vi "change_color_palette_hot_cold_pixels.vi"(8 "error in (no error)":errorcluster, 10 "raw channel index":i32, 11 "DisplayDL090216 in":refnum<class "DisplayDL090216.lvclass">) -> (0 "error out":errorcluster, 3 "DisplayDL090216 out":refnum<class "DisplayDL090216.lvclass">)   [LabVIEW 2010, in "DisplayDL090216.lvclass"]
uses:
  DisplayDL090216.lvclass
  DisplayDL090216.lvclass/DisplayDL090216.ctl
  common/classes/ColorOverlay/ColorOverlay/ColorOverlay.lvclass
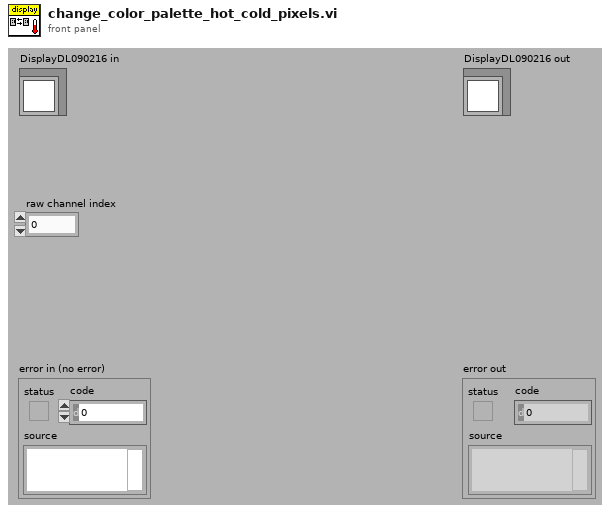
[diagram p1: front panel]
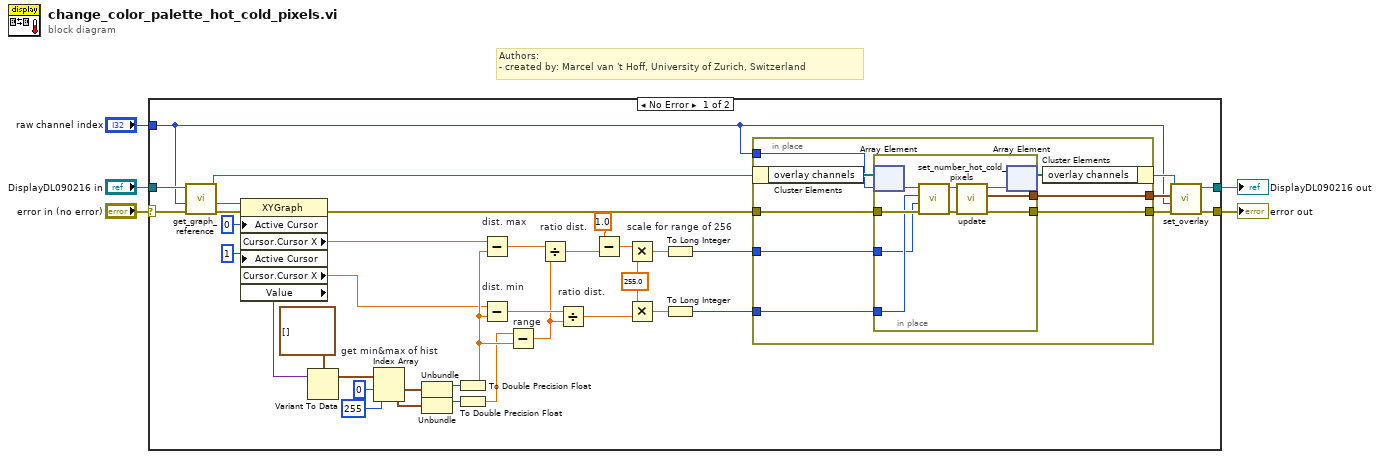
[diagram p0: block diagram]
diagram:
  # "Authors: \n- created by: Marcel van 't Hoff, University of Zurich, Switzerland"
  n1 = case shown="No Error" "error in (no error)" {
    selector: "error in (no error)" -> [w16 w63]
    tunnel: [w6 w63] -> w1
    tunnel: [w7 w62] -> w2
    tunnel: "DisplayDL090216 in" -> [w21 w62]
    tunnel: "raw channel index" -> [w8 _]
    frame No Error {
      w40 = 255.0
      n2 = call-dynamic "get_graph_reference.vi"("error in (no error)"=w16, "raw channel index"=w8, "DisplayDL090216 in"=w21) -> ("error out"=w20:errorcluster, "histogram reference out"=w19:refnum<vi>, "DisplayDL090216 out"=w10:refnum<class "DisplayDL090216.lvclass">)  [unwired: 6 in]
      n3 = property class="XYGraph"(reference=w19, error in=w20, "Active Cursor"=u32 0, "Active Cursor"=u32 1) -> (error out=w15:errorcluster, "Cursor.Cursor X"=w13:dbl, "Cursor.Cursor X"=w14:dbl, "Value"=w35:variant)  [unwired: 1 out]
      n4 = Variant To Data(Variant=w35, type=cluster{i32, u32}[] [] ("histogram out")) -> (data=w34:cluster{i32, u32}[])  [unwired: 1 in, 1 out]
      n5 = Index Array "get min&max of hist"(array=w34, index #1=0 ("index"), index #2=255 ("index")) -> (element #1=w33:cluster{i32, u32}, element #2=w32:cluster{i32, u32})
      n6 = Unbundle(w33) -> (w29:i32)  [unwired: 1 out]
      n7 = Unbundle(w32) -> (w28:i32)  [unwired: 1 out]
      n8 = To Double Precision Float(number=w29) -> (double precision float=w27:dbl)
      n9 = To Double Precision Float(number=w28) -> (double precision float=w26:dbl)
      n10 = Subtract "dist. max"(x=w13, y=w27) -> (x-y=w43:dbl)
      n11 = Subtract "dist. min"(x=w14, y=w27) -> (x-y=w44:dbl)
      n12 = Subtract "range"(x=w26, y=w27) -> (x-y=w42:dbl)
      n13 = Divide "ratio dist."(x=w43, y=w42) -> (x/y=w38:dbl)
      n14 = Divide "ratio dist."(x=w44, y=w42) -> (x/y=w41:dbl)
      n15 = Subtract(x=1.0, y=w38) -> (x-y=w37:dbl)
      n16 = Multiply "scale for range of 256"(x=w37, y=w40) -> (x*y=w23:dbl)
      n17 = Multiply(x=w40, y=w41) -> (x*y=w22:dbl)
      n18 = To Long Integer(number=w23) -> (32bit integer=w11:i32)
      n19 = To Long Integer(number=w22) -> (32bit integer=w12:i32)
      n20 = in-place {
        in-place-border: [w52] -> w18
        in-place-border: w8 -> [w46]
        in-place-border: [w51] -> w17
        in-place-border: w15 -> [w50]
        in-place-border: w12 -> [w49]
        in-place-border: w11 -> [w48]
        n21 = in-place-cluster #1(w10) -> ("overlay channels"=w47:refnum<class "ColorOverlay.lvclass">[])
        n22 = in-place {
          in-place-border: [w61] -> w52
          in-place-border: [w60] -> w51
          in-place-border: w50 -> [w57]
          in-place-border: w49 -> [w56]
          in-place-border: w48 -> [w55]
          n23 = in-place-array #2(w47, w46) -> (w54:refnum<class "ColorOverlay.lvclass">)
          n24 = call-dynamic "set_number_hot_cold_pixels.vi"("error in (no error)"=w57, "# hot pixels"=w55, "# cold pixels"=w56, "ColorOverlay in"=w54) -> ("error out"=w58:errorcluster, "ColorOverlay out"=w59:refnum<class "ColorOverlay.lvclass">)  [unwired: 6 in]
          n25 = call-dynamic "update.vi"("error in (no error)"=w58, "ColorOverlay in"=w59) -> ("error out"=w61:errorcluster, "color cluster out"=w60:cluster{"Red":u8, "Green":u8, "Blue":u8}[], "ColorOverlay out"=w53:refnum<class "ColorOverlay.lvclass">)  [unwired: 7 in]
          n26 = in-place-array #2(w53) -> (w45:refnum<class "ColorOverlay.lvclass">[])  [unwired: 1 out]
        }
        n27 = in-place-cluster #1("overlay channels"=w45) -> (w9:refnum<class "DisplayDL090216.lvclass">)
      }
      n28 = call-dynamic "set_overlay.vi"("error in (no error)"=w18, "raw channel index"=w8, "palette in"=w17, "DisplayDL090216 in"=w9) -> ("error out"=w6:errorcluster, "DisplayDL090216 out"=w7:refnum<class "DisplayDL090216.lvclass">)  [unwired: 6 in]
    }
    frame Error {
    }
  }
  "error out" <- w1
  "DisplayDL090216 out" <- w2
